vi "Requires CLFN Processing.vi"(11 "Manifestation Writer In":refnum<class "Manifestation Writer.lvclass">) -> (2 "Requires Processing?":bool, 3 "Manifestation Writer Out":refnum<class "Manifestation Writer.lvclass">)   [LabVIEW 2013, in "Manifestation Writer.lvclass"]
doc: "This VI should return TRUE if a value of the Writer's type must undergo some kind of processing before being wired to/from a CLFN.\n\nThis VI should return FALSE if a value the Writer's type can be wired directly to/from a CLFN.\n\nThe default implementation returns FALSE.\n\nCopyright (c) 2016 Sze Howe Koh\n\nThis Source Code Form is subject to the terms of the Mozilla Public License, v. 2.0. If a copy of the MPL was not distributed with this file, You can obtain one at http://mozilla.org/MPL/2.0/."
uses:
  Manifestation Writer.lvclass
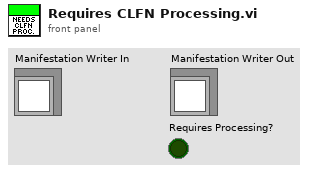
[diagram p1: front panel]
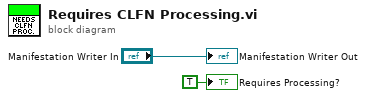
[diagram p0: block diagram]
diagram:
  "Manifestation Writer Out" <- "Manifestation Writer In"
  "Requires Processing?" <- TRUE ("Requires Processing?")
